vi "Post-Build Action.vi"(4 "measurement plugin service":refnum<class "Measurement Plugin Service.lvclass">, 5 "files generated by build":path[](array[path]), 6 "top level/always included VIs":path[](array[path]), 7 "destination path":path, 8 "error in":errorcluster, 9 "target name":string, 10 "build specification name":string, 11 "project path":path) -> (0 "error out":errorcluster)   [LabVIEW 2021, in "NI Measurement Plug-In SDK.lvlib"]
uses:
  NI Measurement Plug-In SDK.lvlib
  Measurement Plugin Service/Measurement Plugin Service.lvclass
  <vilib>/Utility/config.llb/Write Key (String).vi
  <vilib>/Utility/config.llb/NI_LVConfig.lvlib
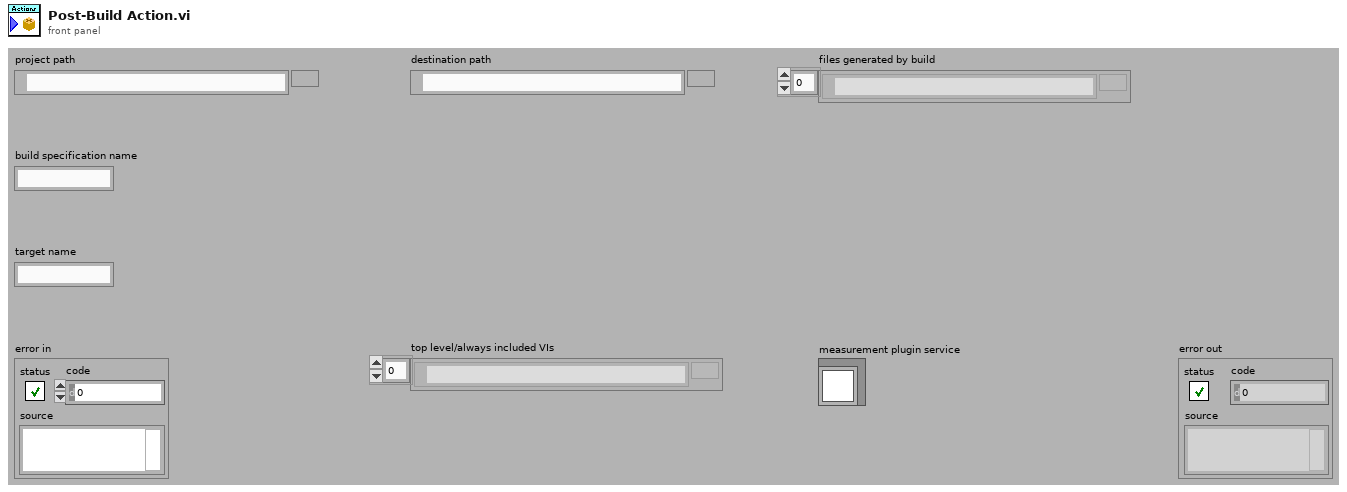
[diagram p1: front panel]
types:
  T1 = cluster{"target name":string, "top level/always included VIs":path[], "project path":path, "destination path":path, "build specification name":string, "files generated by build":path[]}
  T2 = typedef "NI Measurement Plug-In SDK.lvlib/User Interface Details.ctl" = cluster{"file url":string}
  T3 = typedef "NI Measurement Plug-In SDK.lvlib/Measurement Details.ctl" = cluster{"display name":string, "version":string}
  T4 = typedef "NI Measurement Plug-In SDK.lvlib/Measurement Annotation.ctl" = cluster{"key":string, "value":string}
  T5 = typedef "NI_LVConfig.lvlib/Config Data RefNum.ctl" = refnum<k1>
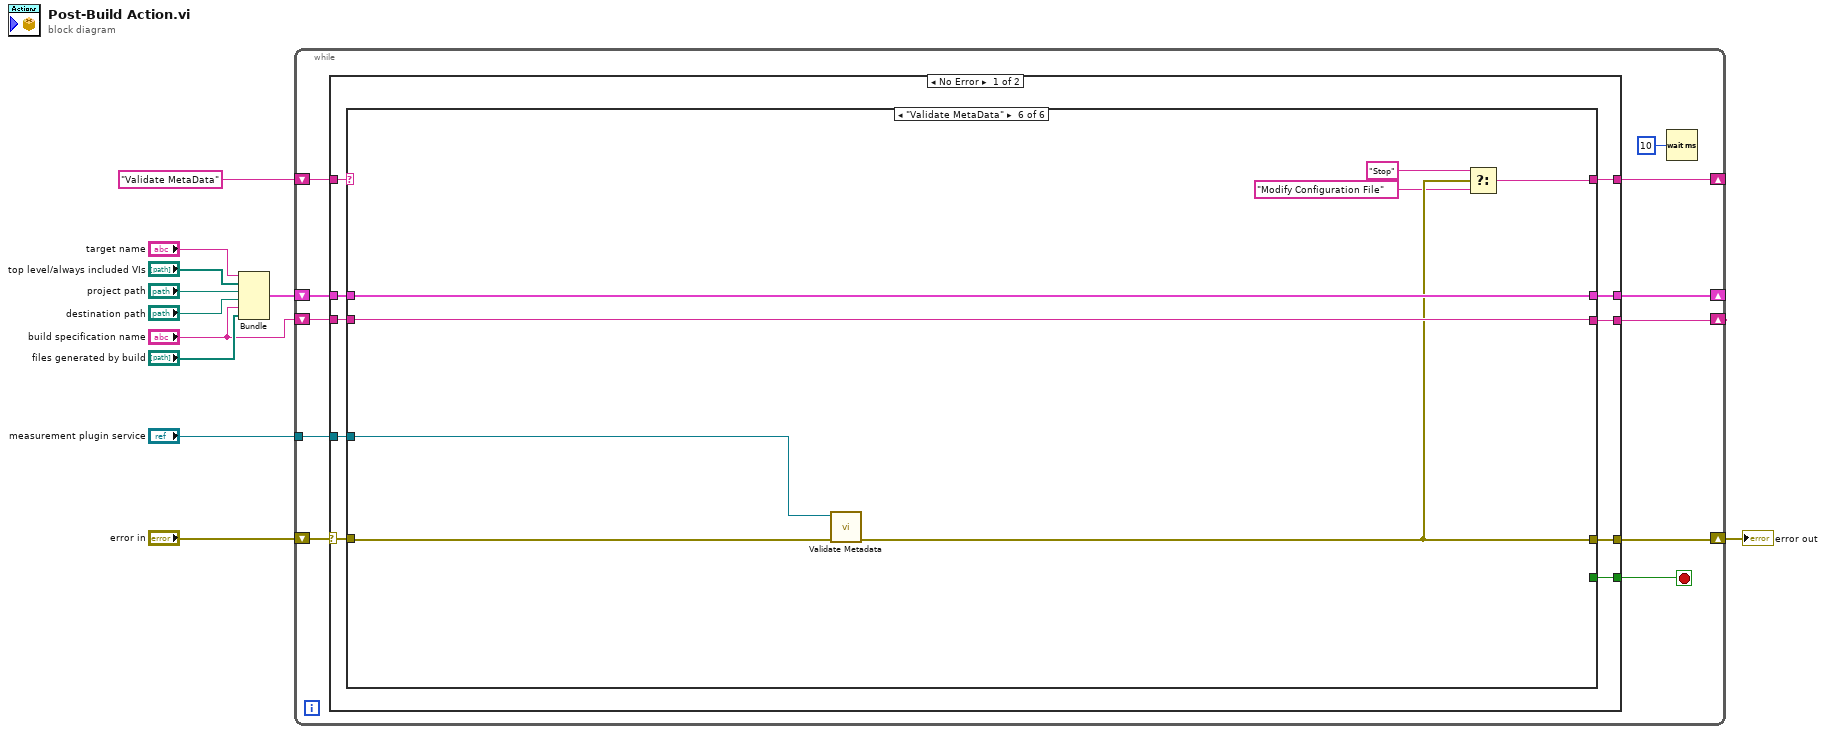
[diagram p0: block diagram]
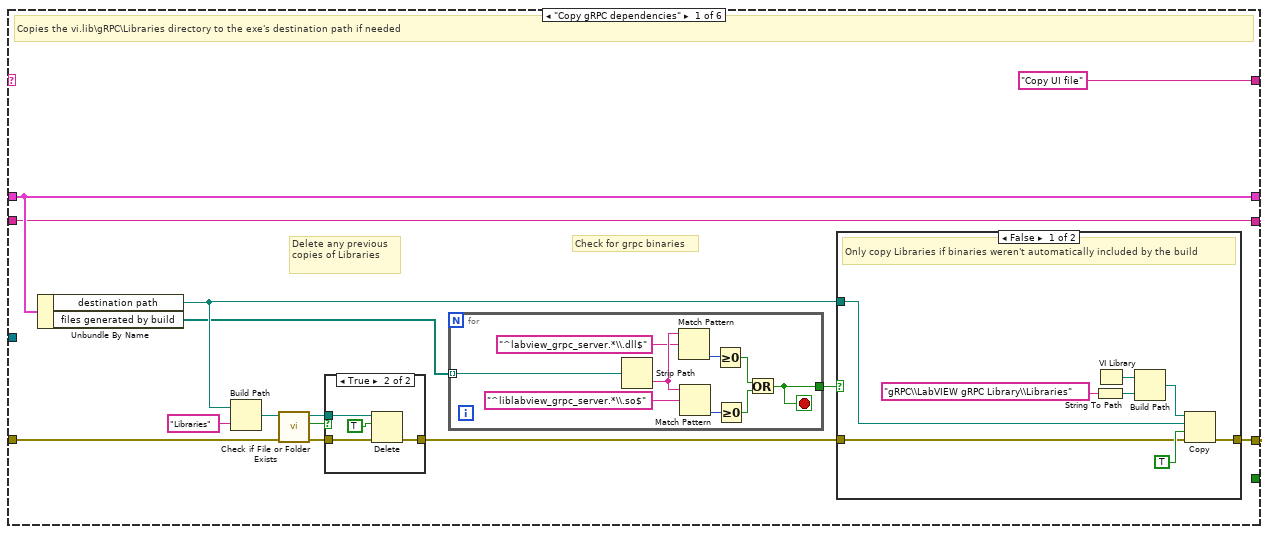
[diagram p2: hidden frame]
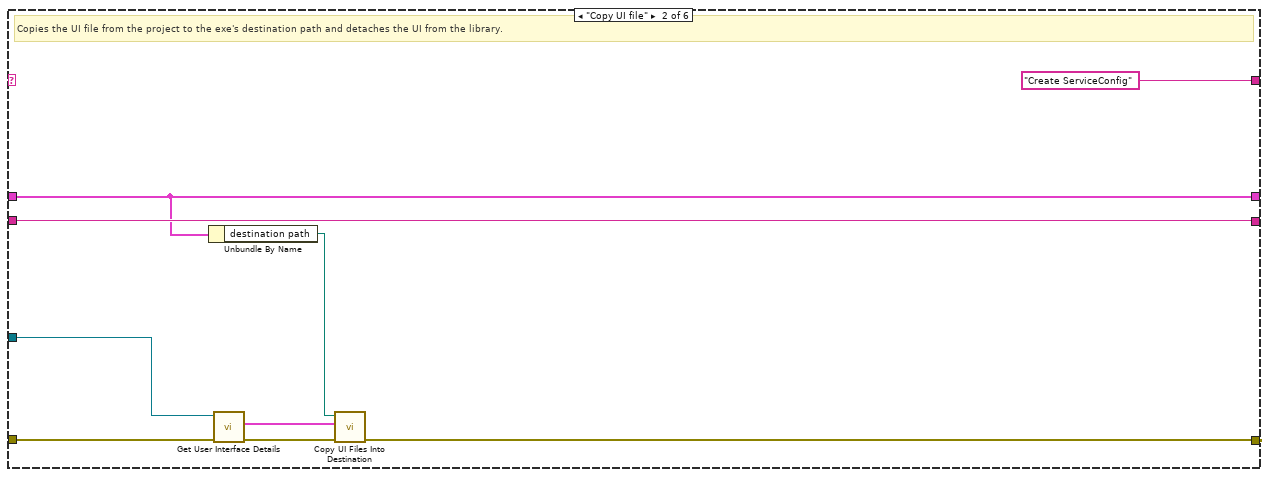
[diagram p5: hidden frame]
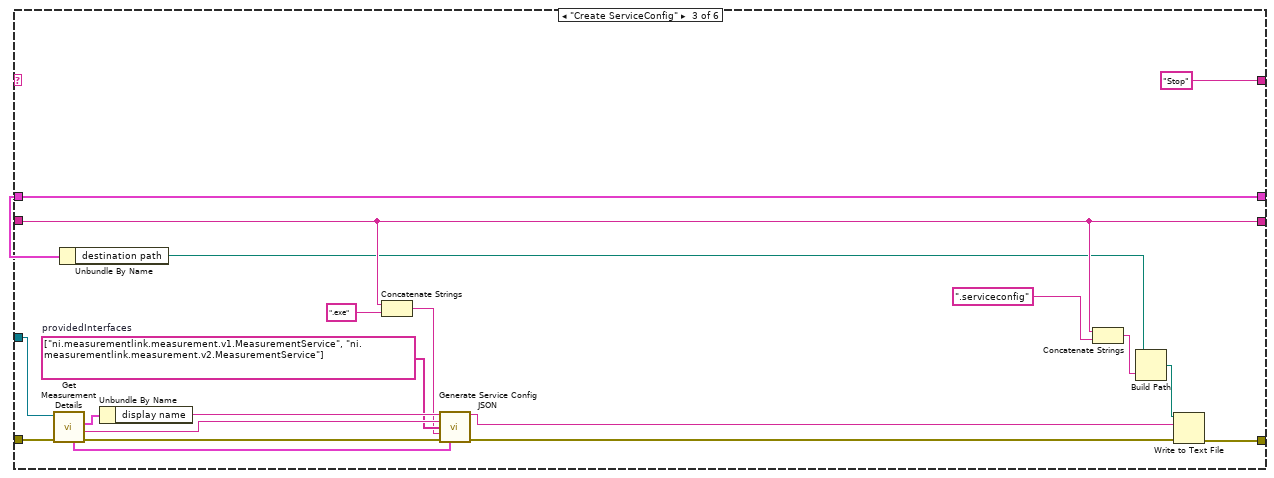
[diagram p6: hidden frame]
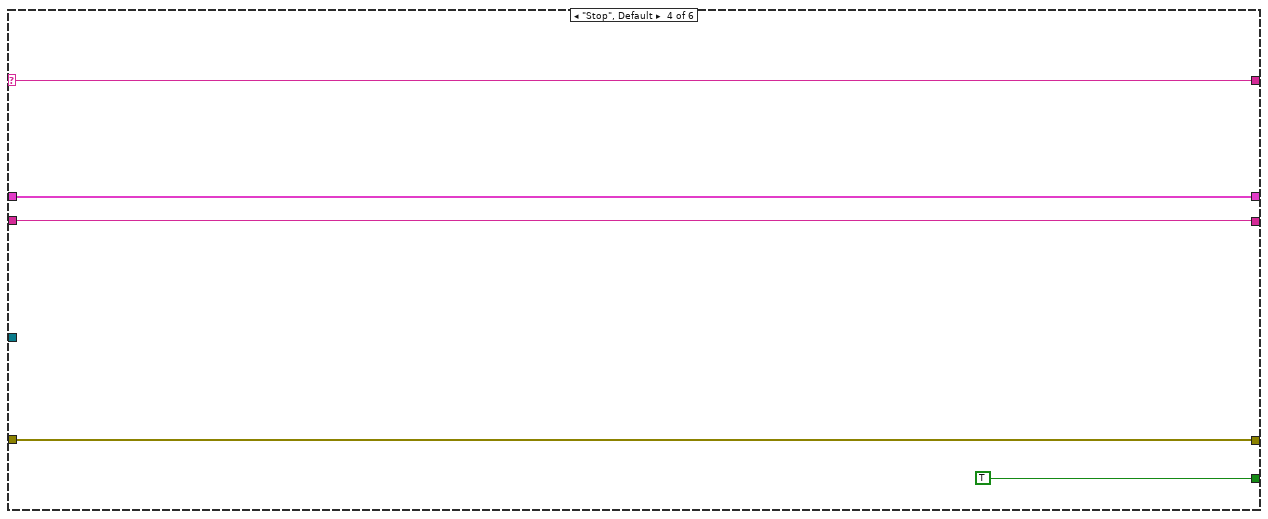
[diagram p7: hidden frame]
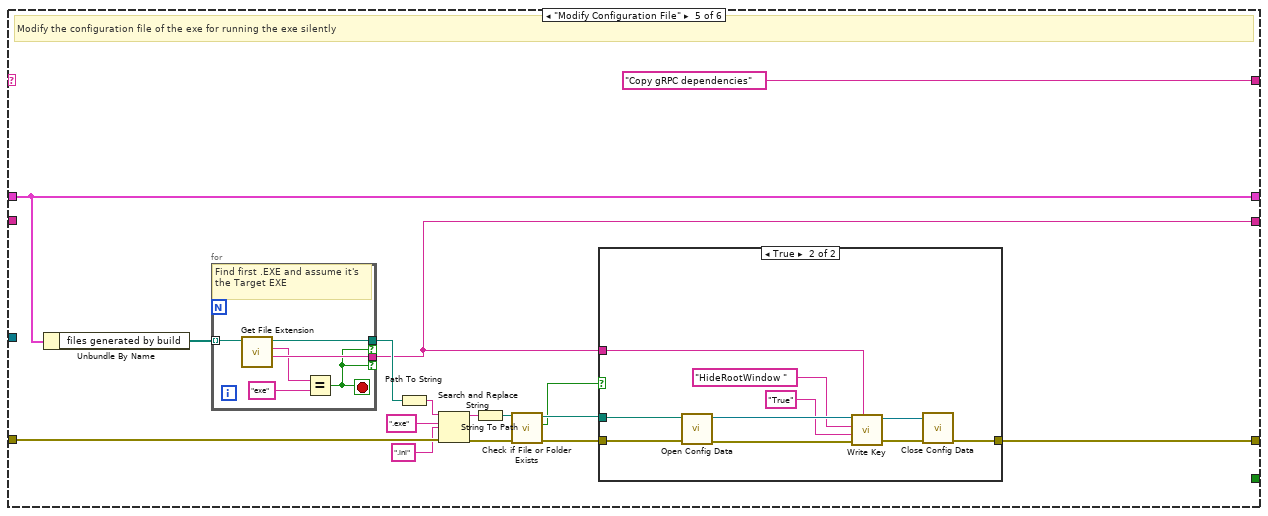
[diagram p8: hidden frame]
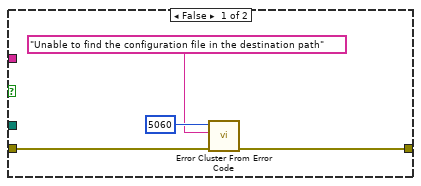
[diagram p9: hidden frame]
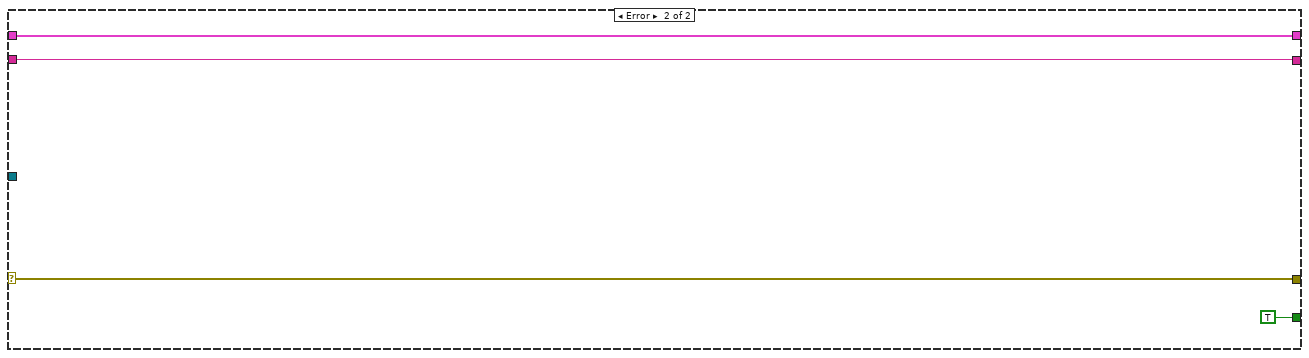
[diagram p10: hidden frame]
diagram:
  n1 = Bundle("target name"="target name", "top level/always included VIs"="top level/always included VIs", "project path"="project path", "destination path"="destination path", "build specification name"="build specification name", "files generated by build"="files generated by build") -> (w5:T1)  [unwired: 1 in]
  n2 = while {
    shift-right: [w19] -> _
    shift-left: w5 -> [w20]
    shift-right: [w18] -> w3
    shift-left: "error in" -> [w15]
    shift-right: [w17] -> _
    shift-left: "Validate MetaData" -> [w21]
    shift-right: [w14] -> _
    shift-left: "build specification name" -> [w13]
    tunnel: "measurement plugin service" -> [w12]
    stop <- w16 stop-if-true
    n3 = case shown="No Error" w15 {
      selector: w15 -> [w26 w150]
      tunnel: w21 -> [w32 _]
      tunnel: w20 -> [w31 w151]
      tunnel: [w30 w151] -> w19
      tunnel: [w29 w150] -> w18
      tunnel: [w28 _] -> w17
      tunnel: [w27 TRUE] -> w16
      tunnel: [w25 w148] -> w14
      tunnel: w13 -> [w24 w148]
      tunnel: w12 -> [w23 _]
      frame No Error {
        n4 = case shown="\"Validate MetaData\"" w32 {
          selector: w32 -> [_ _ _ w101 _ _]
          tunnel: w31 -> [w44 w75 w98 w103 w115 w147]
          tunnel: [w44 w75 w98 w103 w115 w147] -> w30
          tunnel: w26 -> [w36 w73 w88 w100 w113 w145]
          tunnel: [w46 w74 w91 w100 w119 w143] -> w29
          tunnel: ["Copy UI file" "Create ServiceConfig" "Stop" w101 "Copy gRPC dependencies" w140] -> w28
          tunnel: [_ _ _ TRUE _ _] -> w27
          tunnel: [w43 w77 w95 w99 w105 w146] -> w25
          tunnel: w24 -> [w43 w77 w95 w99 _ w146]
          tunnel: w23 -> [_ w71 w89 _ _ w144]
          frame "Copy gRPC dependencies" {
            # "Delete any previous copies of Libraries"
            # "Check for grpc binaries"
            # "Copies the vi.lib\\gRPC\\Libraries directory to the exe's destination path if needed"
            n5 = Unbundle By Name(w44) -> ("destination path"=w35:path, "files generated by build"=w33:path[])
            n6 = Build Path(base path=w35, name or relative path="Libraries") -> (appended path=w41:path)
            n7 = call <vilib>:"Check if File or Folder Exists.vi"("error in (no error)"=w36, "path"=w41) -> ("error out"=w40:errorcluster, "file or folder exists?"=w38:bool, "dup path"=w39:path)  [unwired: 7 in]
            n8 = case shown="True" w38 {
              tunnel: w40 -> [w56 w60]
              tunnel: [w56 w59] -> w34
              tunnel: w39 -> [_ w57]
              frame False {
              }
              frame True {
                n9 = Delete(path (use dialog)=w57, entire hierarchy (F)=TRUE ("confirm (F)"), error in=w60) -> (error out=w59:errorcluster)  [unwired: 2 in, 2 out]
              }
            }
            n10 = for {
              tunnel: [w47] -> w42
              tunnel: w33 -> [w52] mode=indexing
              stop <- w47 stop-if-true
              n11 = Strip Path(path=w52) -> (name=w55:string)  [unwired: 1 out]
              n12 = Match Pattern(string=w55, regular expression="^labview_grpc_server.*\\.dll$" ("pattern")) -> (offset past match=w51:i32)  [unwired: 1 in, 3 out]
              n13 = Match Pattern(string=w55, regular expression="^liblabview_grpc_server.*\\.so$" ("pattern")) -> (offset past match=w50:i32)  [unwired: 1 in, 3 out]
              n14 = Greater Or Equal To 0?(x=w51) -> (x >= 0?=w49:bool)
              n15 = Greater Or Equal To 0?(x=w50) -> (x >= 0?=w48:bool)
              n16 = Or(x=w49, y=w48) -> (x .or. y?=w47:bool)
            }
            n17 = case shown="False" w42 {
              tunnel: [w64 w69] -> w46
              tunnel: w35 -> [w62 _]
              tunnel: w34 -> [w61 w69]
              frame False {
                # "Only copy Libraries if binaries weren't automatically included by the build"
                n18 = String To Path(string="gRPC\\LabVIEW gRPC Library\\Libraries") -> (path=w66:path)
                n19 = VI Library() -> (path=w68:path)
                n20 = Build Path(base path=w68, name or relative path=w66) -> (appended path=w65:path)
                n21 = Copy(8:w61, 9:TRUE ("overwrite (F)"), 10:w62, 11:w65) -> (0:w64:errorcluster)  [unwired: 1 in, 2 out]
              }
              frame True {
              }
            }
          }
          frame "Copy UI file" {
            # "Copies the UI file from the project to the exe's destination path and detaches the UI from the library."
            n22 = Unbundle By Name(w75) -> ("destination path"=w76:path)
            n23 = call-dynamic "Get User Interface Details.vi"("error in"=w73, "measurement plugin service in"=w71) -> ("error out"=w72:errorcluster, "user interface details"=w70:T2[])  [unwired: 7 in, 1 out]
            n24 = call "Copy UI Files Into Destination.vi"("error in"=w72, "user interface details"=w70, "destination path"=w76) -> ("error out"=w74:errorcluster)  [unwired: 8 in]
          }
          frame "Create ServiceConfig" {
            w83 = string[] ["ni.measurementlink.measurement.v1.MeasurementService", "ni.measurementlink.measurement.v2.MeasurementService"]  # providedInterfaces
            n25 = call-dynamic "Get Measurement Details.vi"("error in"=w88, "measurement plugin service in"=w89) -> ("error out"=w86:errorcluster, "service class"=w84:string, "measurement details"=w87:T3, "measurement annotations"=w81:T4[])  [unwired: 5 in, 1 out]
            n26 = Unbundle By Name(w98) -> ("destination path"=w93:path)
            n27 = Unbundle By Name(w87) -> ("display name"=w85:string)
            n28 = Concatenate Strings(w95, ".exe" ("string")) -> (w82:string)
            n29 = call "Generate Service Config JSON.vi"("display name"=w85, "service class"=w84, "provided interfaces"=w83, "path"=w82, "error in"=w86, "annotations"=w81) -> ("service config JSON"=w79:string, "error out"=w80:errorcluster)  [unwired: 8 in]
            n30 = Concatenate Strings(w95, ".serviceconfig" ("string")) -> (w92:string)
            n31 = Build Path(base path=w93, name or relative path=w92) -> (appended path=w90:path)
            n32 = Write to Text File(file (use dialog)=w90, text=w79, error in=w80) -> (error out=w91:errorcluster)  [unwired: 1 in, 2 out]
          }
          frame "Stop", Default {
          }
          frame "Modify Configuration File" {
            # "Modify the configuration file of the exe for running the exe silently"
            n33 = Unbundle By Name(w115) -> ("files generated by build"=w114:path[])
            n34 = for {
              tunnel: w114 -> [w125] mode=indexing
              tunnel: [w124] -> w105 if=w120
              tunnel: [w123] -> w107 if=w120
              stop <- w120 stop-if-true
              # "Find first .EXE and assume it's the Target EXE"
              n35 = call <vilib>:"Get File Extension.vi"("file"=w125) -> ("filename without extension"=w124:string, "lowercase file extension"=w121:string, "dup file"=w123:path)  [unwired: 6 in, 2 out]
              n36 = Equal?(x=w121, y="exe") -> (x = y?=w120:bool)
            }
            n37 = Path To String(path=w107) -> (string=w106:string)
            n38 = Search and Replace String(input string=w106, search string=".exe", replace string=".ini", error in=w113) -> (result string=w110:string, error out=w112:errorcluster)  [unwired: 4 in, 2 out]
            n39 = String To Path(string=w110) -> (path=w109:path)
            n40 = call <vilib>:"Check if File or Folder Exists.vi"("error in (no error)"=w112, "path"=w109) -> ("error out"=w118:errorcluster, "file or folder exists?"=w116:bool, "dup path"=w117:path)  [unwired: 7 in]
            n41 = case shown="True" w116 {
              tunnel: [w128 w139] -> w119
              tunnel: w117 -> [_ w132]
              tunnel: w118 -> [w129 w131]
              tunnel: w105 -> [_ w130]
              frame False {
                n42 = call <vilib>:"Error Cluster From Error Code.vi"("error in (no error)"=w129, "error message (\"\")"="Unable to find the configuration file in the destination path" ("source"), "error code (0)"=5060) -> ("error out"=w128:errorcluster)  [unwired: 6 in]
              }
              frame True {
                n43 = call <vilib>:"Open Config Data.vi"("error in (no error)"=w131, "configuration file path"=w132) -> ("error out"=w138:errorcluster, "refnum"=w137:T5)  [unwired: 7 in, 1 out]
                n44 = call-poly <vilib>:"Write Key.vi"("section"=w130, "error in (no error)"=w138, "value"="True", "key"="HideRootWindow ", "refnum"=w137) -> ("error out"=w135:errorcluster, "refnum out"=w134:T5)  [unwired: 4 in, 1 out]
                n45 = call <vilib>:"Close Config Data.vi"("error in (no error)"=w135, "refnum"=w134) -> ("error out"=w139:errorcluster)  [unwired: 8 in, 1 out]
              }
            }
          }
          frame "Validate MetaData" {
            n46 = call "Validate Metadata.vi"("error in"=w145, "measurement plugin service in"=w144) -> ("error out"=w143:errorcluster)  [unwired: 8 in, 1 out]
            n47 = Select(t="Stop", s=w143, f="Modify Configuration File") -> (s? t:f=w140:string)
          }
        }
      }
      frame Error {
      }
    }
    n48 = Wait (ms)(milliseconds to wait=u32 10 ("millisecond timer value")) -> ()  [unwired: 1 out]
  }
  "error out" <- w3
